vi "Init.vi"(11 "UI Refs":T1) -> (0 "Error Out":errorcluster)   [LabVIEW 2015, in "SB SubVIs.lvlib"]
uses:
  SB SubVIs.lvlib
  Type Defs/UI Refs.ctl
  Type Defs/Dashboard.ctl
  Type Defs/Square Cluster.ctl
  Square/Square.lvclass
  Globals.vi
  Endigit Library/Endigit.lvlib
  Type Defs/SB Type Defs.lvlib
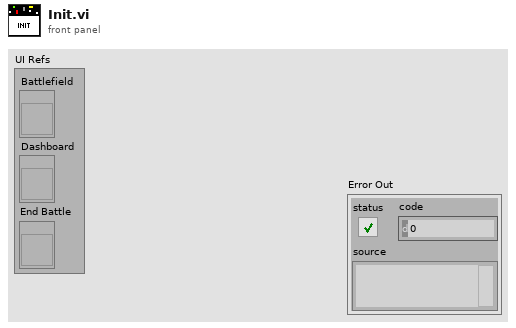
[diagram p1: front panel]
types:
  T1 = typedef "SB Type Defs.lvlib/UI Refs.ctl" = cluster{"Battlefield":refnum<vi>, "Dashboard":refnum<vi>, "End Battle":refnum<vi>}
  T2 = typedef "SB Type Defs.lvlib/Dashboard.ctl" = cluster{"Color":u32, "Player":i32, "Status":string, "Stats":string}
  T3 = typedef "SB Type Defs.lvlib/Square Cluster.ctl" = cluster{"Attacked":bool, "Team":i32, "Next Turn":i32, "DVR":refnum<data-value>}
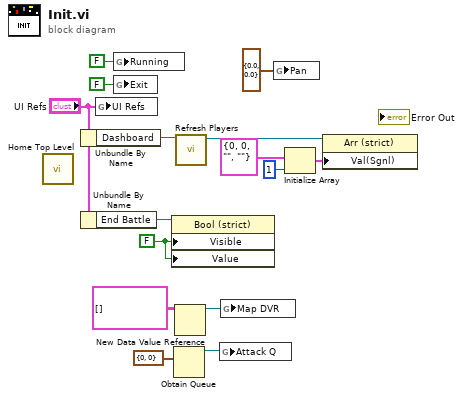
[diagram p0: block diagram]
diagram:
  w11 = FALSE ("Visible")
  n1 = call "Home Top Level.vi"() -> ()  [unwired: 11 in]
  n2 = Unbundle By Name("UI Refs") -> ("Dashboard"=w5:refnum<vi>)
  n3 = Unbundle By Name("UI Refs") -> ("End Battle"=w12:refnum<vi>)
  n4 = global write "Globals.vi" "UI Refs"("UI Refs") -> ()
  n5 = global write "Globals.vi" "Running"(FALSE ("Exit")) -> ()
  n6 = global write "Globals.vi" "Exit"(FALSE ("Exit")) -> ()
  n7 = property on="Property Node" class="Bool (strict)"(reference=w12, "Visible"=w11, "Value"=w11) -> ()  [unwired: 1 in, 2 out]
  n8 = Obtain Queue(element data type=cluster{"Row":i32, "Column":i32} {"Row"=0, "Column"=0} ("output cluster")) -> (queue out=w2:refnum<queue>)  [unwired: 4 in, 2 out]
  n9 = New Data Value Reference(data value=T3[][] [] ("initialized array")) -> (data value reference=w13:refnum<data-value>)  [unwired: 1 in, 1 out]
  n10 = call "Refresh Players.vi"("Dashboard"=w5) -> ("Dashboard"=w4:refnum<vi>)  [unwired: 10 in]
  n11 = global write "Globals.vi" "Attack Q"(w2) -> ()
  n12 = global write "Globals.vi" "Map DVR"(w13) -> ()
  n13 = global write "Globals.vi" "Pan"(cluster{"Horizontal":dbl, "Vertical":dbl} {"Horizontal"=0.0, "Vertical"=0.0} ("Pan")) -> ()
  n14 = Initialize Array(T2 {"Color"=0, "Player"=0, "Status"="", "Stats"=""} ("Dashboard"), 1 ("dimension size")) -> (w7:T2[])
  n15 = property class="Arr (strict)"(reference=w4, "Val(Sgnl)"=w7) -> ()  [unwired: 1 in, 2 out]
